vi "Start.vi"(0 "reference in":refnum<class "niMmWave_Transceiver.lvclass">, 5 "TX bursts":refnum<class "mmWave data.lvclass">[](array[class]), 7 "sequence":string[](array[string]), 9 "RX acq duration":dbl=320000.0, 11 "error in (no error)":errorcluster) -> (4 "reference out":refnum<class "niMmWave_Transceiver.lvclass">, 15 "error out":errorcluster)   [LabVIEW 2019, in "niMmWave_Transceiver.lvclass"]
doc: "Starts insturment operation:"
uses:
  niMmWave_Transceiver.lvclass
  C:/Barkhausen mmWave radar/Development/modules/mmw_instrument/src_LabVIEW/Host/SubVIs/mmWave instrument_class/mmWave instrument.lvclass
  mmWave data_class/mmWave data.lvclass
  mmWave instrument_class/Instrument state.ctl
  BurstInfo.ctl
  mmWave HW Control/HW custom error.ctl
  58af3c7a-4da3-4af3-b250-a184b4a370b4.vi
  <vilib>/addons/Modulation/Analog/MT Resample (Complex Cluster).vi
  <vilib>/addons/Modulation/Analog/support/Validators/mod_Fractional Resample Validate.vi
  <vilib>/addons/Modulation/Analog/support/Validators/mod_Check Flush State.vi
  <vilib>/addons/Modulation/Analog/support/mod_FractionalResampler.vi
  <vilib>/addons/Modulation/Analog/support/mod_Integer Rate Interpolation.vi
  <vilib>/addons/Modulation/Analog/support/mod_Set Error Source.vi
  <vilib>/addons/Modulation/Analog/support/Validators/mod_Validate Complex Waveform.vi
  <vilib>/addons/Modulation/Analog/support/mod_PerformResampling.vi
  <vilib>/addons/Modulation/Analog/support/Validators/mod_WFErrorHandler.vi
  <vilib>/Utility/error.llb/Error Cluster From Error Code.vi
  <vilib>/addons/Modulation/Analog/support/mod_Resampling Factors.vi
  <vilib>/addons/Modulation/Analog/support/mod_ResamplingFilter.vi
  <vilib>/addons/Modulation/Analog/support/mod_Generate Integer Interpolation Filter.vi
  mmWave instrument_class/mmWave instrument.lvclass
  mmWave HW Control/mmWave HW Control.lvlib
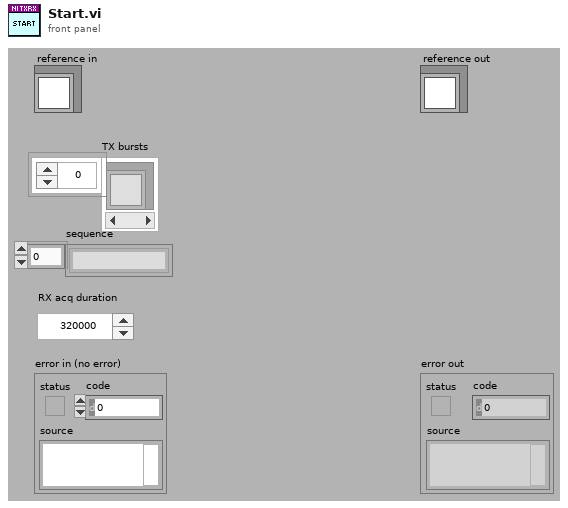
[diagram p1: front panel]
types:
  T1 = typedef "mmWave instrument.lvclass/Instrument state.ctl" = enum16{"Off", "Initialization", "Configuration", "Running", "Calibration"}
  T2 = typedef "niMmWave_Transceiver.lvclass/BurstInfo.ctl" = cluster{"starting addr":u32, "end addr":u32}
  T3 = typedef "mmWave instrument.lvclass/ObjectAttributes.ctl" = cluster{"mode":T4, "instr state":T1, "Max Fs":dbl, "Equalization coeff":cdb[], "LO sync en":bool, "Trig sync en":bool, "LO sources":T5, "LO Export":T6, "Fc.range":cluster{"min":dbl, "max":dbl}, "Sync mode":T7, "equalization en":bool, "sequence":string[]}
  T4 = typedef "mmWave instrument.lvclass/Instrument mode.ctl" = enum16{"RF", "IF", "BB"}
  T5 = typedef "mmWave HW Control.lvlib/LO sources.ctl" = cluster{"RX/LO1 src":string, "TX/LO1 src":string, "LO2 src":string}
  T6 = typedef "mmWave HW Control.lvlib/LO export.ctl" = cluster{"TX LO1 export":bool, "TX LO1 export level":dbl, "RX LO1 export":bool, "RX LO1 export level":dbl, "LO2 export":bool, "LO2 export level":dbl}
  T7 = typedef "mmWave instrument.lvclass/Sync mode.ctl" = enum16{"Slave", "Master"}
  T8 = typedef "niMmWave_Transceiver.lvclass/ObjectAttributesRef.ctl" = refnum<data-value>
  T9 = typedef "niMmWave_Transceiver.lvclass/ObjectAttributes.ctl" = cluster{"session":T10[], "HW.RX resources":T24, "RF config":T25, "RX trigger options":T26, "TX trigger options":T26, "RX samples":i32, "Downloaded Bursts":map{string, T2}, "TX Fs":dbl, "RX Fs":dbl, "burst sequence":string[]}
  T10 = typedef "Session.ctl" = cluster{"3620 session":refnum<queue>, "tx baseband session":T11, "rx baseband session":T19, "tx gain (dB)":dbl, "rx gain (dB)":dbl, "hardware configuration":T20, "gain ranging":T22[], "pxi trigger bus information":T23}
  T11 = typedef "Tx Baseband Session.ctl" = cluster{"3610 session":T12, "7902 reference":T18}
  T12 = typedef "ni3610_and_ni3630_Driver_Lib.lvlib/Main Settings.ctl" = cluster{"VISA resource name":refnum<visa-resource-name>, "Address Space":T13, "window_offset":u32, "register_addresses":T14, "required_MM_fpga_version":cluster{"signature":u32, "hardware":u32, "current revision":u32, "oldest revision":u32}, "CPLD Oldest Compat Version ":cluster{"hardware":u32, "CPLD firmware":u32}, "MM_FPGA_image_location":string, "is_init":bool, "card_type":T15, "DacLmkConfigFileName":string, "AdcLmkConfigFileName":string, "AdcConfigFileName":string, "DacConfigFileName_RevA":string, "DacConfigFileName_RevB":string, "Mulde hardware revision":u8, "bypass DAC PLL\n":bool, "IQ Card Revision":T16, "board capability":T17}
  T13 = typedef "VISA Register Access Address Space.ctl" = u16
  T14 = typedef "ni3610_and_ni3630_Driver_Lib.lvlib/Register Adresses.ctl" = cluster{"MM based Registers":cluster{"Revision":u32, "OldestCompatRev":u32, "signature":u32, "scratch":u32, "LedControl":u32, "BoardHwRev":u32, "BoardControl":u32, "ThermalStatus":u32, "BasebandStatus":u32, "BasebandControl":u32, "BasebandAuxSetup":u32, "BasebandAuxStatus":u32, "LmkSyncOutSetup":u32, " AdcSyncOutSetup":u32, " InjSyncOutSetup":u32, " PxiTrig0OutSetup":u32, " PxiTrig1OutSetup":u32, " PxiTrig2OutSetup":u32, " PxiTrig3OutSetup":u32, " PxiTrig4OutSetup":u32, " PxiTrig5OutSetup":u32, " PxiTrig6OutSetup":u32, " PxiTrig7OutSetup":u32}, "CPLD based Registers":cluster{"SlaveSignature":u32, "SlaveRevision":u32, "SlaveOldestCompatRev":u32, "SlaveScratch":u32, "SlaveSetup":u32, "SlaveStatus":u32, "IDacReg_offset":u32, "LMKRegGrp0_offset":u32, "QDacReg_offset":u32, "BrdTempSensorVal":u32, "TempSensorPowerDown":u32, "GPIOReg_offset":u32, "IAdcReg_offset":u32, "QAdcReg_offset":u32, "LMKRegGrp1_offset":u32, "QadcTempSensorVal":u32, "IadcTempSensorVal":u32, "RevisionReg":u32, "VcxoReg":u32, "CpldStatusReg":u32, "PowerReg":u32, "VBiasEnReg":u32, "ExtRefOeReg":u32, "QdacCtrlReg":u32, "QdacStatusReg":u32, "IdacCtrlReg":u32, "IdacStatusReg":u32, "QdacJtagIn":u32, "QdacJtagOut":u32, "IdacJtagIn":u32, "IdacJtagOut":u32, "IqDcSetupReg":u32, "QadcStatusReg":u32, "IadcStatusReg":u32, "BrdSetupReg":u32, "IqDcRevisionReg":u32, "PllStatusReg":u32, "EndpointScratchReg":u32, "AdcSyncCfgReg":u32, "IqCardOpampReg":u32}, "CPLD Register Offset":u32, "MM  Register Offset":u32, " PxiTrig0OutSetup":u32}
  T15 = typedef "ni3610_and_ni3630_Driver_Lib.lvlib/Base Card Type.ctl" = enum16{"unspecified", "ADC", "DAC"}
  T16 = typedef "ni3610_and_ni3630_Driver_Lib.lvlib/IQ Card Revision.ctl" = enum16{"RevA", "RevB", "RevC", "RevD"}
  T17 = typedef "ni3610_and_ni3630_Driver_Lib.lvlib/Board Capability.ctl" = cluster{"baseband sync":enum16{"no baseband sync", "baseband sync"}}
  T18 = typedef "Blank FPGA Reference.ctl" = refnum<k20>
  T19 = typedef "Rx Baseband Session.ctl" = cluster{"3630 session":T12, "7902 reference":T18}
  T20 = typedef "Hardware Configuration.ctl" = cluster{"direction":T21, "baseband only":bool}
  T21 = typedef "Direction.ctl" = enum16{"Transceiver", "Receiver", "Transmitter"}
  T22 = typedef "Gain Ranging.ctl" = cluster{"gain ranging active scope":string, "gain ranging stream session":refnum<k20>}
  T23 = typedef "PXI Trigger Bus Info.ctl" = cluster{"chassis resource name":refnum<visa-resource-name>, "7902R (TX)":i16, "3610 (TX)":i16, "3620 (IF)":i16, "3630 (RX)":i16, "7902R (RX)":i16}
  T24 = typedef "mmWave HW Control.lvlib/HW TXRX resources cluster.ctl" = cluster{"TX_DAC":refnum<visa-resource-name>, "TX_FPGA":tag, "IF":tag, "RX_ADC":refnum<visa-resource-name>, "RX_FPGA":tag}
  T25 = typedef "mmWave HW Control.lvlib/HW TXRX RF config cluster.ctl" = cluster{"TX.Frequency":dbl, "TX.Gain":dbl, "TX.mmWave adapter":string, "RX.Frequency":dbl, "RX.Gain":dbl, "RX.mmWave adapter":string}
  T26 = typedef "TX trigger config.ctl" = cluster{"delay":dbl, "trig source":T27, "PXI src":i32, "export":T28, "PXI dest":i32}
  T27 = typedef "FPGA Utility.lvlib/FPGA driver trigger source.ctl" = enum16{"Use Tclk", "PXI_Trig", "Aurora RX trig"}
  T28 = typedef "FPGA Utility.lvlib/FPGA driver trigger destination.ctl" = enum16{"None", "Source trig", "Synced trig", "Delayed sync"}
  T29 = typedef "mmWave HW Control.lvlib/HW custom error.ctl" = u16
  T30 = typedef "Constants.ctl" = cluster{"data clock rate (Hz)":dbl, "sample rate (Hz)":dbl, "sample rate selector string":string, "default tx bitfile path":path, "default rx bitfile path":path, "default proc bitfile path":path}
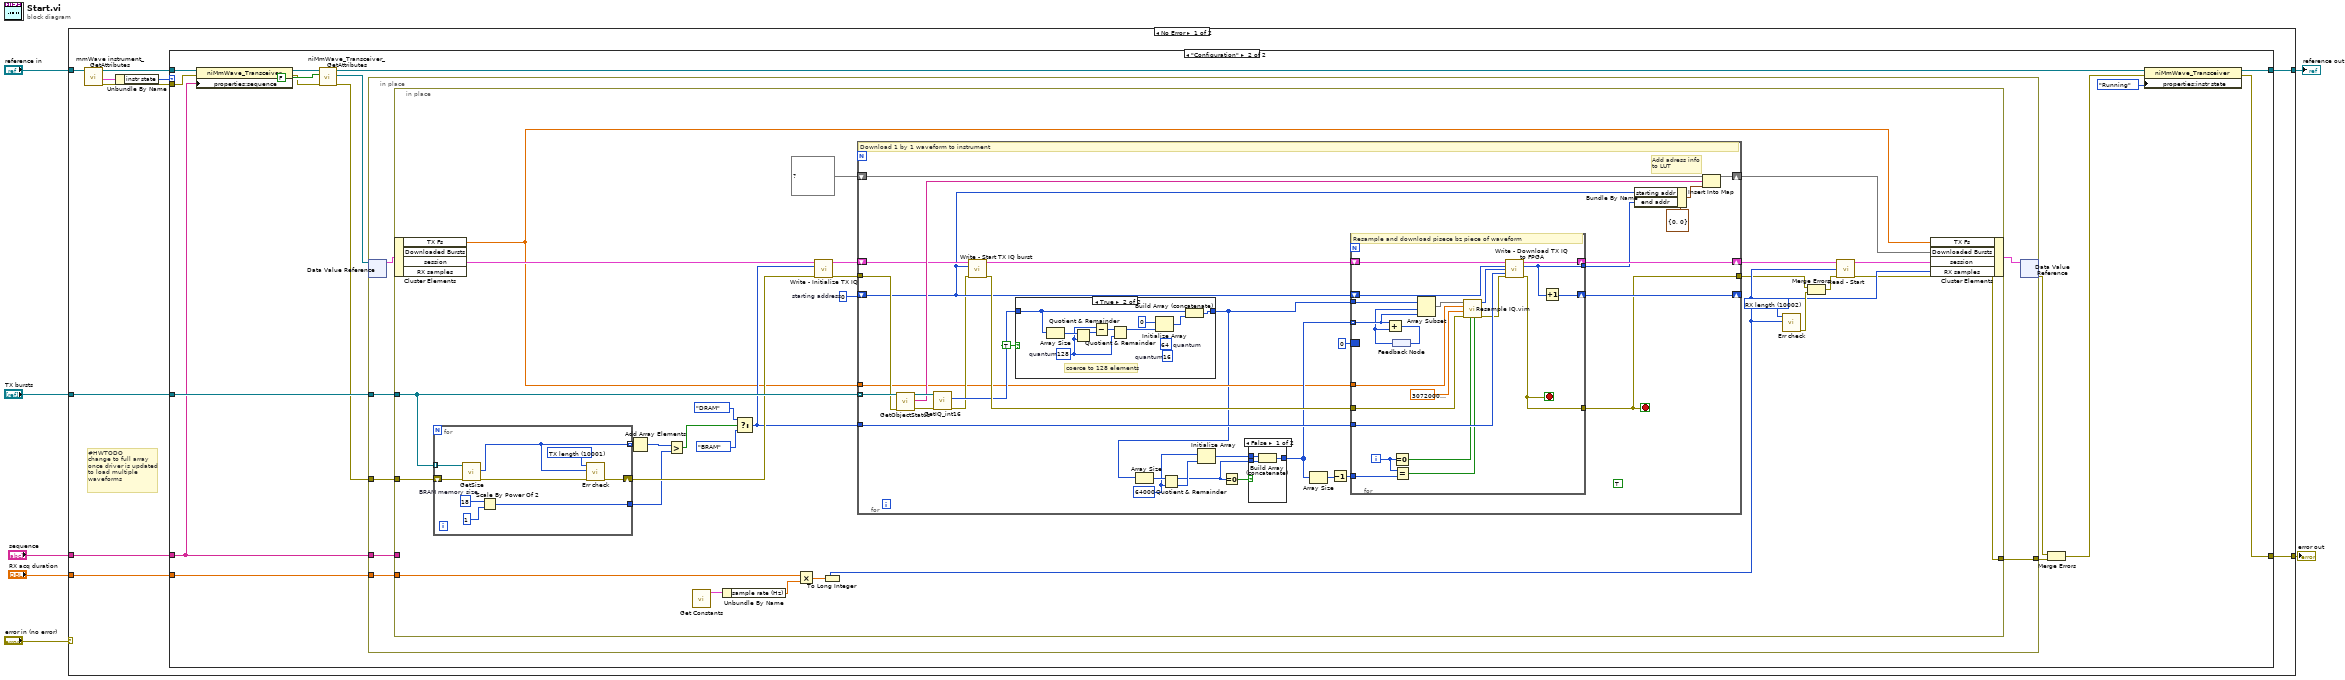
[diagram p0: block diagram]
diagram:
  n1 = case shown="No Error" "error in (no error)" {
    selector: "error in (no error)" -> [_ w150]
    tunnel: [w17 w150] -> w6
    tunnel: [w15 w149] -> w4
    tunnel: "reference in" -> [w16 w149]
    tunnel: "TX bursts" -> [w9 _]
    tunnel: "RX acq duration" -> [w10 _]
    tunnel: "sequence" -> [w8 _]
    frame No Error {
      # "#HWTODO\nchange to full array\nonce driver is updated\nto load multiple\nwaveforms"
      n2 = call "mmWave instrument_GetAttributes.vi"("reference in"=w16) -> ("error out"=w11:errorcluster, "attributes"=w13:T3, "reference out"=w14:refnum<class "niMmWave_Transceiver.lvclass">)  [unwired: 7 in, 1 out]
      n3 = Unbundle By Name(w13) -> ("instr state"=w12:T1)
      n4 = case shown="\"Configuration\"" w12 {
        tunnel: [_ w24] -> w17
        tunnel: [w18 w27] -> w15
        tunnel: w14 -> [w18 w23]
        tunnel: w9 -> [_ w31]
        tunnel: w11 -> [_ w21]
        tunnel: w10 -> [_ w30]
        tunnel: w8 -> [_ w19]
        frame "Off", Default {
        }
        frame "Configuration" {
          n5 = property class="niMmWave_Transceiver"(reference=w23, error in=w21, "properties:sequence"=w19) -> (reference out=w22:refnum<class "niMmWave_Transceiver.lvclass">, error out=w20:errorcluster)
          n6 = call "niMmWave_Transceiver_GetAttributes.vi"("error in (no error)"=w20, "return data? (T)"=FALSE, "reference in"=w22) -> ("error out"=w29:errorcluster, "attributes ref"=w32:T8, "reference out"=w33:refnum<class "niMmWave_Transceiver.lvclass">)  [unwired: 5 in, 1 out]
          n7 = in-place {
            in-place-border: w31 -> [w40]
            in-place-border: w30 -> [w39]
            in-place-border: w29 -> [w38]
            in-place-border: [w37] -> w28
            in-place-border: w19 -> [w36]
            n8 = in-place-dvr #1(w32) -> (w41:T9)  [unwired: 1 out]
            n9 = in-place {
              in-place-border: w40 -> [w69]
              in-place-border: w39 -> [w53]
              in-place-border: w38 -> [w66]
              in-place-border: [w49] -> w37
              in-place-border: w36 -> [_]
              w64 = T29 10002 items=["TX list"=10000, "TX length"=10001, "RX length"=10002] ("HW custom err")
              w68 = u32 0  # starting address
              n10 = in-place-cluster #2(w41) -> ("TX Fs"=w54:dbl, "session"=w61:T10[])  [unwired: 2 out]
              n11 = for {
                tunnel: w69 -> [w148] mode=indexing
                shift-right: [w142] -> w59
                shift-left: w66 -> [w145]
                tunnel: [w141] -> w46
                tunnel: [w140] -> w45 mode=indexing
                w144 = T29 10001 items=["TX list"=10000, "TX length"=10001, "RX length"=10002] ("HW custom err")
                w146 = i16 18  # BRAM memory size
                n12 = call-dynamic "GetSize.vi"("error in (no error)"=w145, "reference in"=w148) -> ("error out"=w143:errorcluster, "Size"=w140:i32)  [unwired: 6 in, 2 out]
                n13 = Scale By Power Of 2(n=w146, x=1) -> (x*2^n=w141:i32)
                n14 = call "Err check.vi"("error in"=w143, "Variant Control"=w140, "HW custom err"=w144) -> ("error out"=w142:errorcluster)  [unwired: 8 in]
              }
              n15 = Add Array Elements(numeric array=w45) -> (sum=w44:i32)
              n16 = Greater?(x=w44, y=w46) -> (0:w43:bool)
              n17 = call "Get Constants.vi"() -> ("constants"=w48:T30)  [unwired: 15 in]
              n18 = Unbundle By Name(w48) -> ("sample rate (Hz)"=w47:dbl)
              n19 = Select(t=enum16{"DRAM", "BRAM"}."DRAM" ("burst memo 2"), s=w43, f=enum16{"DRAM", "BRAM"}."BRAM" ("burst memo 2")) -> (s? t:f=w58:enum16{"DRAM", "BRAM"})
              n20 = Multiply(x=w53, y=w47) -> (x*y=w55:dbl)
              n21 = call "Write - Initialize TX IQ.vi"("session in"=w61, "memo"=w58, "error in"=w59) -> ("session out"=w60:T10[], "error out"=w57:errorcluster)  [unwired: 11 in]
              n22 = To Long Integer(number=w55) -> (32bit integer=w52:i32)
              n23 = for {
                shift-right: [w90] -> w67
                shift-left: w60 -> [w94]
                tunnel: w69 -> [w101] mode=indexing
                shift-right: [w104] -> _
                shift-left: w68 -> [w91]
                tunnel: w57 -> [w95]
                shift-right: [w103] -> w56
                shift-left: map{string, T2} {} ("Downloaded Bursts") -> [w102]
                tunnel: w54 -> [w73]
                tunnel: w58 -> [w89]
                tunnel: [w74] -> w51
                stop <- w74 stop-if-true
                w85 = 64000 ("y")
                (unwired) TRUE ("zero pad")
                # "Add adress info\nto LUT"
                # "Download 1 by 1 waveform to instrument"
                n24 = call-dynamic "GetObjectStatus.vi"("reference in"=w101, "error in (no error)"=w95) -> ("reference out"=w100:refnum<class "mmWave data.lvclass">, "object name"=w99:string, "error out"=w96:errorcluster)  [unwired: 6 in, 9 out]
                n25 = call-dynamic "GetIQ_int16.vi"("error in (no error)"=w96, "reference in"=w100) -> ("error out"=w75:errorcluster, "data"=w76:i16[])  [unwired: 6 in, 2 out]
                n26 = call "Write - Start TX IQ burst.vi"("session in"=w94, "Wfm addr"=w91, "error in"=w75) -> ("session out"=w93:T10[], "error out"=w92:errorcluster)  [unwired: 11 in]
                n27 = case shown="True" TRUE ("zero pad") {
                  tunnel: w76 -> [w126 w131]
                  tunnel: [w126 w130] -> w72
                  frame False {
                  }
                  frame True {
                    (unwired) 64  # quantum
                    w127 = 128  # quantum
                    (unwired) 16  # quantum
                    # "coerce to 128 elements"
                    n28 = Array Size(array=w131) -> (size(s)=w135:i32)
                    n29 = Quotient & Remainder(x=w135, y=w127) -> (x-y*floor(x/y)=w134:i32)  [unwired: 1 out]
                    n30 = Subtract(x=w127, y=w134) -> (x-y=w129:i32)
                    n31 = Quotient & Remainder(x=w129, y=w127) -> (x-y*floor(x/y)=w128:i32)  [unwired: 1 out]
                    n32 = Initialize Array(i16 0 ("element"), w128) -> (w133:i16[])
                    n33 = Build Array (concatenate)(w131, w133) -> (w130:i16[])
                  }
                }
                n34 = Array Size(array=w72) -> (size(s)=w87:i32)
                n35 = Quotient & Remainder(x=w87, y=w85) -> (x-y*floor(x/y)=w83:i32, floor(x/y)=w86:i32)
                n36 = Initialize Array(w85, w86) -> (w84:i32[])
                n37 = Equal To 0?(x=w83) -> (x = 0?=w82:bool)
                n38 = case shown="False" w82 {
                  tunnel: w84 -> [w138 w139]
                  tunnel: [w137 w139] -> w81
                  tunnel: w83 -> [w136 _]
                  frame False {
                    n39 = Build Array (concatenate)(w138, w136) -> (w137:i32[])
                  }
                  frame True {
                  }
                }
                n40 = Array Size(array=w81) -> (size(s)=w80:i32)
                n41 = Decrement(x=w80) -> (x-1=w79:i32)
                n42 = for {
                  tunnel: w73 -> [w122]
                  tunnel: w89 -> [w118]
                  tunnel: w72 -> [w112]
                  tunnel: [w117] -> w88
                  shift-right: [w119] -> w90
                  shift-left: w93 -> [w123]
                  shift-right: [w125] -> w104
                  shift-left: w91 -> [w120]
                  tunnel: w81 -> [w110] mode=indexing
                  tunnel: w79 -> [w114]
                  border: 0 -> [_]
                  tunnel: w92 -> [w107]
                  tunnel: [w105] -> w74
                  i -> [w115]
                  stop <- w105 stop-if-true
                  # "Resample and download pisece bz piece of waveform"
                  n43 = feedback #3() -> (w108:i32)
                  n44 = Add(x=w110, y=w108) -> (x+y=w109:i32)
                  n45 = feedback-in #3(w109) -> ()
                  n46 = Equal To 0?(x=w115) -> (x = 0?=w116:bool)
                  n47 = Equal?(x=w115, y=w114) -> (x = y?=w113:bool)
                  n48 = Array Subset(array=w112, index=w108, length=w110) -> (w111:i16[])
                  n49 = call "Resample IQ.vim"("flush buffers? (T"=w113, "reset? (T)"=w116, "error in (no error)"=w107, "FS out"=3072000000.0, "Fs in"=w122, "data in"=w111) -> ("error out"=w106:errorcluster, "resampled data"=w121:i16[])  [unwired: 4 in]
                  n50 = call "Write - Download TX IQ to FPGA.vi"("session in"=w123, "Wfm addr"=w120, "data"=w121, "memo"=w118, "error in"=w106) -> ("session out"=w119:T10[], "last wr addr"=w117:u32, "error out"=w105:errorcluster)  [unwired: 8 in]
                  n51 = Increment(x=w117) -> (x+1=w125:u32)
                }
                n52 = Bundle By Name(cluster=T2 {"starting addr"=0, "end addr"=0} ("value"), "starting addr"=w91, "end addr"=w88) -> (w97:T2)
                n53 = Insert Into Map(map in=w102, key=w99, value=w97) -> (map out=w103:map{string, T2})  [unwired: 2 out]
              }
              n54 = call "Err check.vi"("Variant Control"=w52, "HW custom err"=w64) -> ("error out"=w63:errorcluster)  [unwired: 9 in]
              n55 = Merge Errors(w51, w63) -> (w50:errorcluster)
              n56 = call "Read - Start.vi"("session in"=w67, "number of samples"=w52, "error in"=w50) -> ("session out"=w62:T10[], "error out"=w49:errorcluster)  [unwired: 11 in]
              n57 = in-place-cluster #2("TX Fs"=w54, "Downloaded Bursts"=w56, "session"=w62, "RX samples"=w52) -> (w42:T9)
            }
            n58 = in-place-dvr #1(w42) -> (w35:errorcluster)  [unwired: 1 out]
          }
          n59 = Merge Errors(w35, w28) -> (w26:errorcluster)
          n60 = property class="niMmWave_Transceiver"(reference=w33, error in=w26, "properties:instr state"=Instrument_state."Running" ("instr state")) -> (reference out=w27:refnum<class "niMmWave_Transceiver.lvclass">, error out=w24:errorcluster)
        }
      }
    }
    frame Error {
    }
  }
  "error out" <- w6
  "reference out" <- w4
